vi "Write Limit Current.vi"(8 "error in":errorcluster, 10 "OverCurrent_Protect":dbl, 11 "36234A in":refnum<class "36234A.lvclass">) -> (0 "error out":errorcluster, 3 "36234A out":refnum<class "36234A.lvclass">)   [LabVIEW 2019, in "36234A.lvlib" / "36234A.lvclass"]
uses:
  Library/36234A.lvclass
  C:/Users/Public/Documents/Development/builds/Instruments/PowerSupply.lvlibp/Library/PowerSupply.lvclass
  Library/36234A.lvclass/36234A.ctl
  builds/Instruments/PowerSupply.lvlibp/Accessors/Read Active Channel.vi
  builds/Instruments/PowerSupply.lvlibp/Library/PowerSupply.lvclass
  <instrlib>/Keysight E36000 Series/Keysight E36000 Series.lvlib
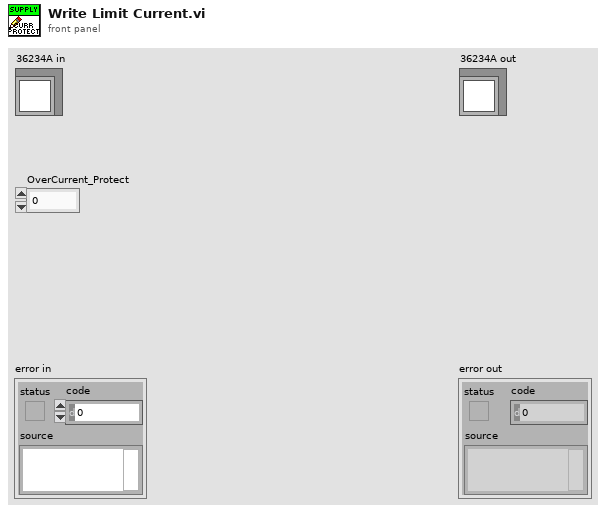
[diagram p1: front panel]
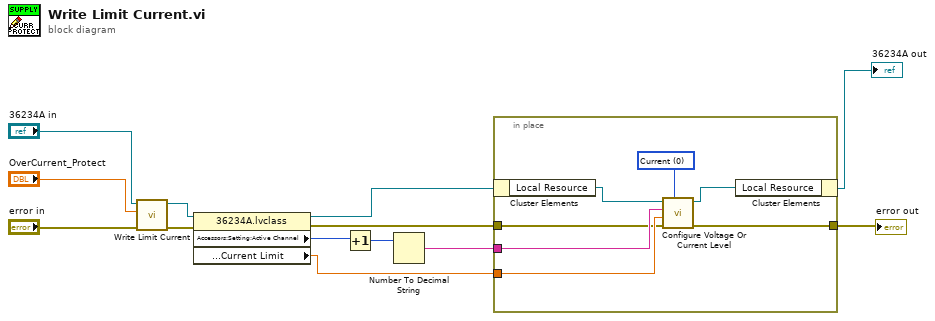
[diagram p0: block diagram]
diagram:
  n1 = call-parent "Write Limit Current.vi"("error in"="error in", "OverCurrent_Protect"="OverCurrent_Protect", "PowerSupply in"="36234A in") -> ("error out"=w10:errorcluster, "PowerSupply out"=w9:refnum<class "36234A.lvclass">)  [unwired: 7 in]
  n2 = property class="36234A.lvclass"(reference=w9, error in=w10) -> (reference out=w5:refnum<class "36234A.lvclass">, error out=w6:errorcluster, "Accessors:Setting:Active Channel"=w2:u32, "Accessors:Setting:Protection:Current Limit"=w1:dbl)
  n3 = Increment(x=w2) -> (x+1=w7:u32)
  n4 = Number To Decimal String(number=w7) -> (decimal integer string=w8:string)  [unwired: 1 in]
  n5 = in-place {
    in-place-border: w8 -> [w17]
    in-place-border: w1 -> [w16]
    in-place-border: w6 -> [w15]
    in-place-border: [w14] -> w3
    w18 = 0 items=["Current", "Voltage"] ("Function (0 : Current)")
    n6 = in-place-cluster #1(w5) -> ("Local Resource"=w20:refnum<visa-resource-name>)
    n7 = call <instrlib>:"Configure Voltage Or Current Level.vi"("Function (0 : Current)"=w18, "error in (no error)"=w15, "Voltage Or Current Level (1)"=w16, "Channel (1)"=w17, "VISA resource name"=w20) -> ("error out"=w14:errorcluster, "VISA resource name out"=w19:refnum<visa-resource-name>)  [unwired: 5 in]
    n8 = in-place-cluster #1("Local Resource"=w19) -> (→"36234A out":refnum<class "36234A.lvclass">)
  }
  "error out" <- w3
